vi "updateVariablesStatus.vi"(8 "error in (no error)":errorcluster, 11 "CoolerControler in":refnum<class "CoolerControler.lvclass">) -> (0 "error out":errorcluster, 3 "CoolerControler out":refnum<class "CoolerControler.lvclass">)   [LabVIEW 2016, in "CoolerControler.lvclass"]
uses:
  CoolerControler.lvclass
  typedefs/readTempreature.ctl
  CoolerControler.lvclass/CoolerControler.ctl
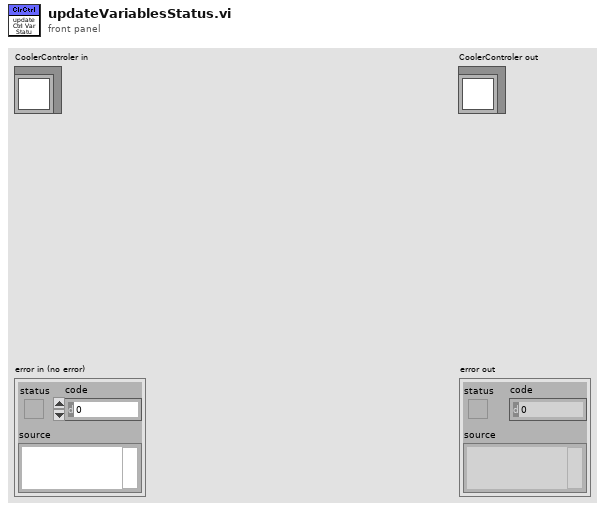
[diagram p1: front panel]
types:
  T1 = typedef "readTempreature.ctl" = enum16{"SetTemperature", "AmbientTemperature", "SupplyTemperature", "ExternalRTDTemperature", "ReturnTemperature", "ExternalThermistor"}
  T2 = typedef "ControlSensor.ctl" = enum16{"SupplyTemperature", "ReturnTemperature", "ExtRTD", "ExternalTermistor"}
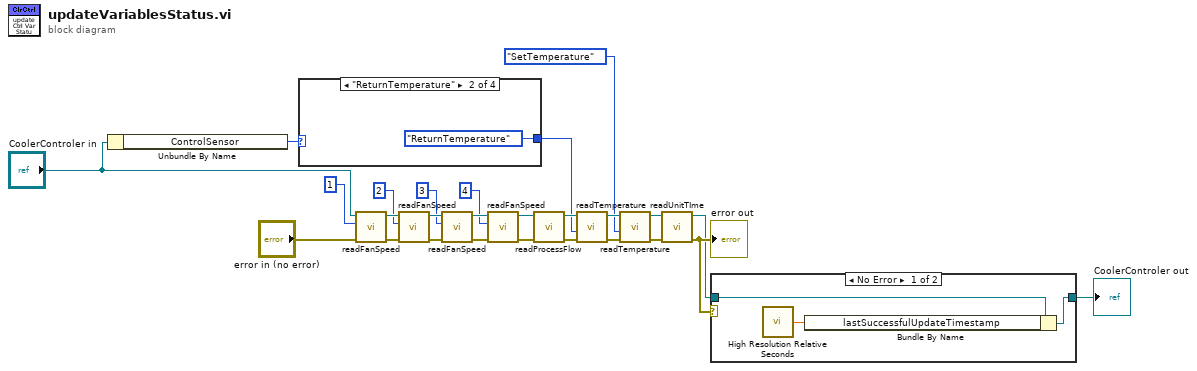
[diagram p0: block diagram]
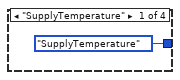
[diagram p2: hidden frame]
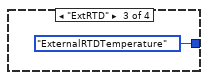
[diagram p3: hidden frame]
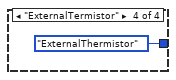
[diagram p4: hidden frame]
diagram:
  n1 = Unbundle By Name("CoolerControler in") -> ("ControlSensor"=w9:T2)
  n2 = case shown="\"ReturnTemperature\"" w9 {
    tunnel: [readTempreature."SupplyTemperature" ("TemperatureType") readTempreature."ReturnTemperature" ("TemperatureType") readTempreature."ExternalRTDTemperature" ("TemperatureType") readTempreature."ExternalThermistor" ("TemperatureType")] -> w8
    frame "SupplyTemperature" {
    }
    frame "ReturnTemperature" {
    }
    frame "ExtRTD" {
    }
    frame "ExternalTermistor" {
    }
  }
  n3 = call "readFanSpeed.vi"("error in (no error)"="error in (no error)", "fanNumber"=1, "CoolerControler in"="CoolerControler in") -> ("error out"=w26:errorcluster, "CoolerControler out"=w25:refnum<class "CoolerControler.lvclass">)  [unwired: 6 in, 1 out]
  n4 = call "readFanSpeed.vi"("error in (no error)"=w26, "fanNumber"=2, "CoolerControler in"=w25) -> ("error out"=w24:errorcluster, "CoolerControler out"=w23:refnum<class "CoolerControler.lvclass">)  [unwired: 6 in, 1 out]
  n5 = call "readFanSpeed.vi"("error in (no error)"=w24, "fanNumber"=3, "CoolerControler in"=w23) -> ("error out"=w22:errorcluster, "CoolerControler out"=w21:refnum<class "CoolerControler.lvclass">)  [unwired: 6 in, 1 out]
  n6 = call "readFanSpeed.vi"("error in (no error)"=w22, "fanNumber"=4, "CoolerControler in"=w21) -> ("error out"=w19:errorcluster, "CoolerControler out"=w20:refnum<class "CoolerControler.lvclass">)  [unwired: 6 in, 1 out]
  n7 = call "readProcessFlow.vi"("error in (no error)"=w19, "CoolerControler in"=w20) -> ("error out"=w15:errorcluster, "CoolerControler out"=w18:refnum<class "CoolerControler.lvclass">)  [unwired: 7 in, 1 out]
  n8 = call "readTemperature.vi"("error in (no error)"=w15, "TemperatureType"=w8, "CoolerControler in"=w18) -> ("error out"=w7:errorcluster, "CoolerControler out"=w6:refnum<class "CoolerControler.lvclass">)  [unwired: 6 in, 1 out]
  n9 = call "readTemperature.vi"("error in (no error)"=w7, "TemperatureType"=readTempreature."SetTemperature", "CoolerControler in"=w6) -> ("error out"=w3:errorcluster, "CoolerControler out"=w4:refnum<class "CoolerControler.lvclass">)  [unwired: 6 in, 1 out]
  n10 = call "readUnitTIme.vi"("error in (no error)"=w3, "CoolerControler in"=w4) -> ("error out"=w2:errorcluster, "CoolerControler out"=w1:refnum<class "CoolerControler.lvclass">)  [unwired: 7 in, 1 out]
  "error out" <- w2
  n11 = case shown="No Error" w2 {
    tunnel: w1 -> [w33 w34]
    tunnel: [w32 w34] -> w17
    frame No Error {
      n12 = call <vilib>:"High Resolution Relative Seconds.vi"() -> ("relative seconds"=w31:dbl)
      n13 = Bundle By Name(cluster=w33, "lastSuccessfulUpdateTimestamp"=w31) -> (w32:refnum<class "CoolerControler.lvclass">)
    }
    frame Error {
    }
  }
  "CoolerControler out" <- w17
